vi "visualizer main.vi"(8 "error in (no error)":errorcluster, 11 "Item Ref in":T3 format="%.0x") -> (0 "error out":errorcluster, 3 "Item Ref out":T3 format="%.0x")   [LabVIEW 2016, in "FPGA RM System Definition API.lvlib"]
uses:
  FPGA RM System Definition API.lvlib
  <vilib>/NI Veristand/Custom Device API/Custom Device Item Ref.ctl
  API/Types/fpga resource.ctl
  API/Types/Channel Type.ctl
  type defs/viz_type.ctl
  type defs/viz_state.ctl
  visualizer globals.vi
  <vilib>/NI VeriStand/Custom Device Tools/Custom Device Utility Library/Custom Device Utility Library.lvlib
  Shared/FPGA RM Shared API.lvlib
  <vilib>/NI VeriStand/Custom Device API/Custom Device API.lvlib
panel:
  out "column width":i32[](array[numeric])
  in  "Options":enum32{"", "Sort", "Filter"}(tab)=enum."Filter"
  in  "Sort By...":T1 items=["RIO device", "resource", "input type", "datatype", "reserver"]
  in  "Datatype":string
  in  "Input Type":T2(ring)
  in  "Resource Name":string
  in  "RIO Device Name":string
  in  "Mappings":i32(listbox)
  in  "Columns":i32(listbox)
  out "mapped and unmapped":bool[](array[boolean])
  out "selected values":bool[](array[boolean])
  in  "table":i32(listbox)
  out "fpga resources":cluster{"fpga cd":T3, "resource":T4}[](array[cluster]) {"fpga cd" format="%.0x"}
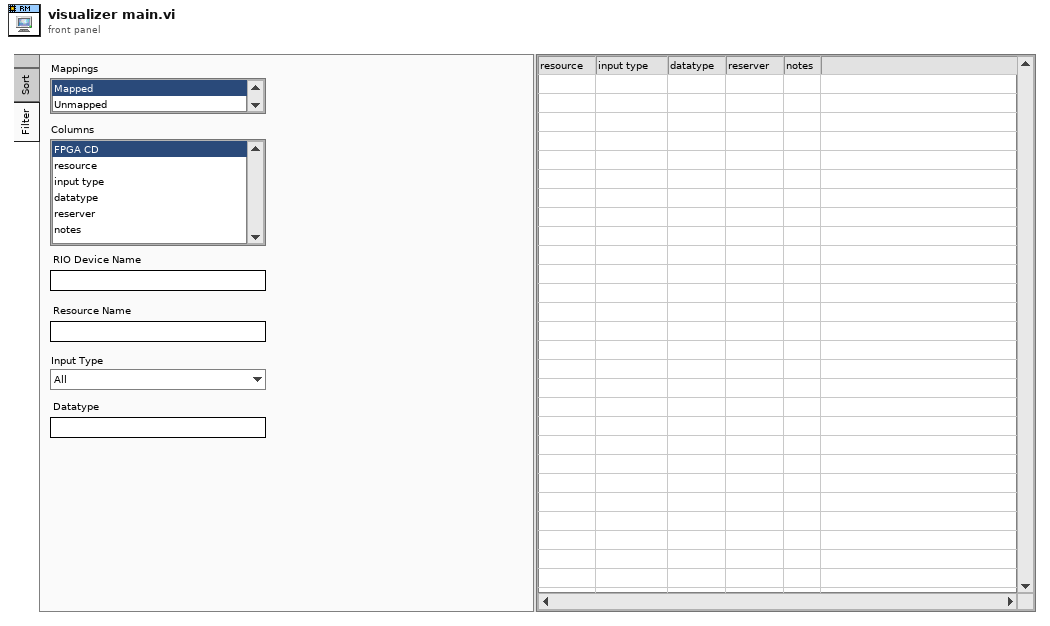
[diagram p1: front panel]
types:
  T1 = typedef "FPGA RM System Definition API.lvlib/viz_type.ctl" = u16
  T2 = enum16{"All", "Write Channel", "Read Channel", "Write Waveform", "Read Waveform"}
  T3 = typedef "Custom Device API.lvlib/Custom Device Item Ref.ctl" = u64
  T4 = typedef "FPGA RM System Definition API.lvlib/fpga resource.ctl" = cluster{"name":string, "datatype":string, "channel type":T5, "value":variant, "notes":string}
  T5 = typedef "FPGA RM System Definition API.lvlib/Channel Type.ctl" = enum16{"Write Channel", "Read Channel", "Write Waveform", "Read Waveform"}
  T6 = typedef "RM.Server.lvlib/viz_command.ctl" = cluster{"state":T7, "data":variant}
  T7 = typedef "RM.Server.lvlib/viz_state.ctl" = enum16{"shutdown"}
  T8 = typedef "FPGA RM System Definition API.lvlib/viz_state.ctl" = enum16{"shutdown"}
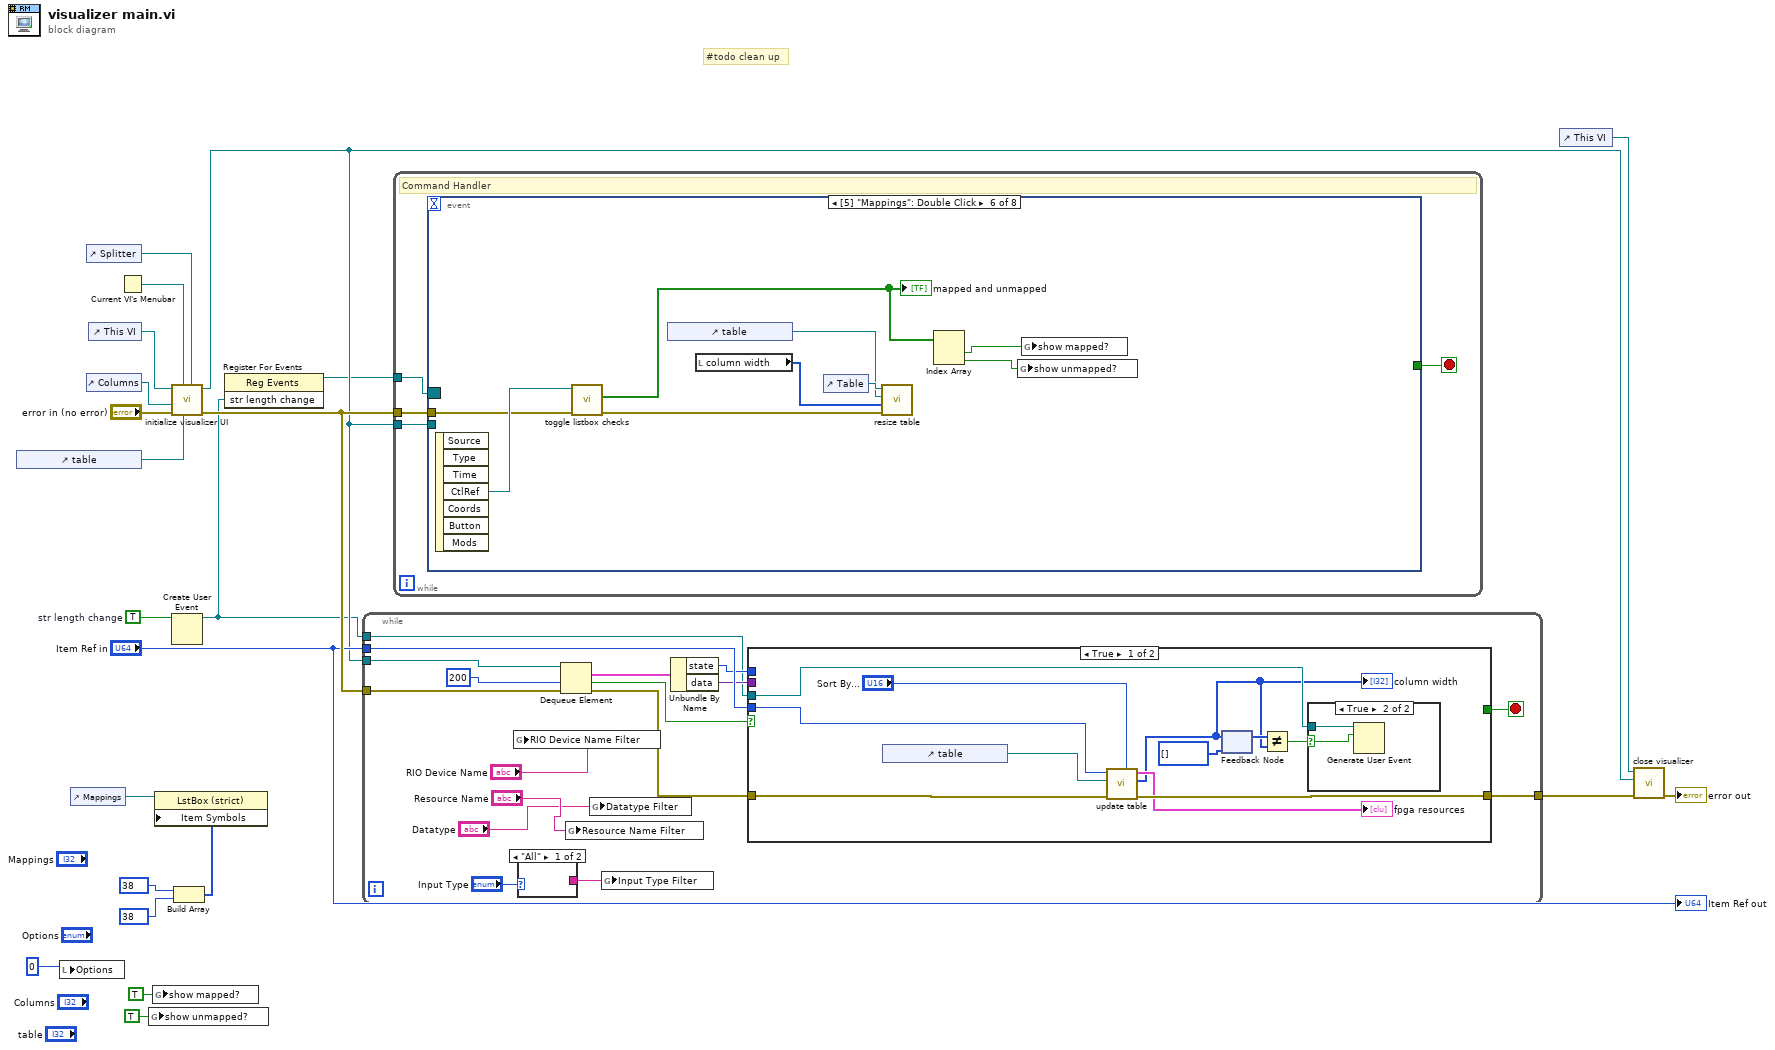
[diagram p0: block diagram]
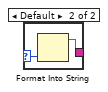
[diagram p2: hidden frame]
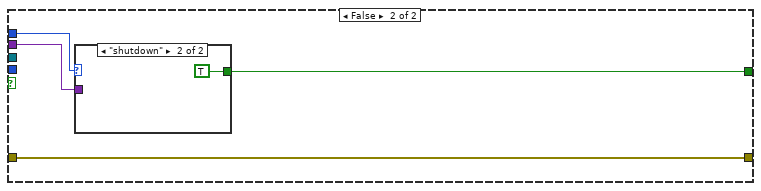
[diagram p4: hidden frame]
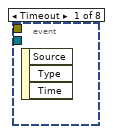
[diagram p6: hidden frame]
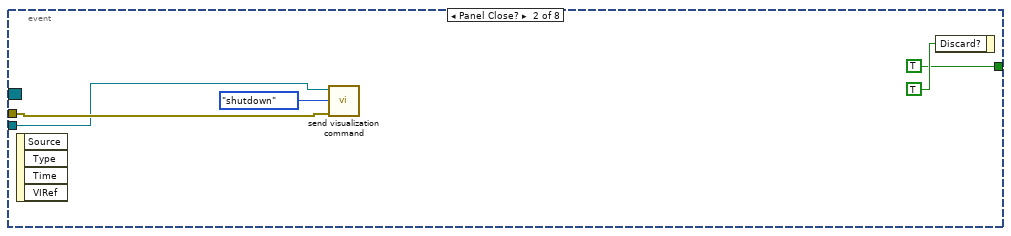
[diagram p7: hidden frame]
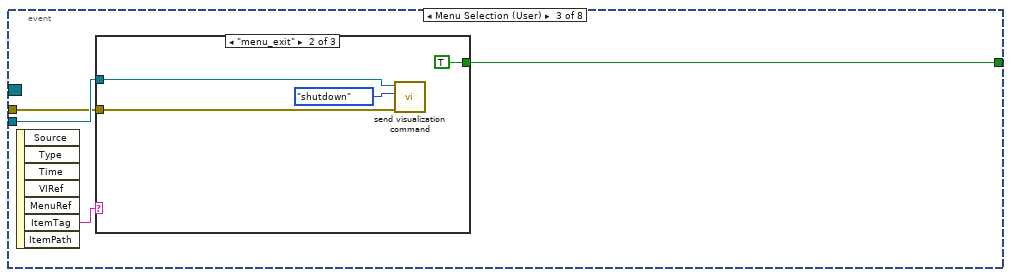
[diagram p8: hidden frame]
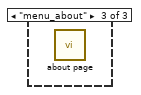
[diagram p10: hidden frame]
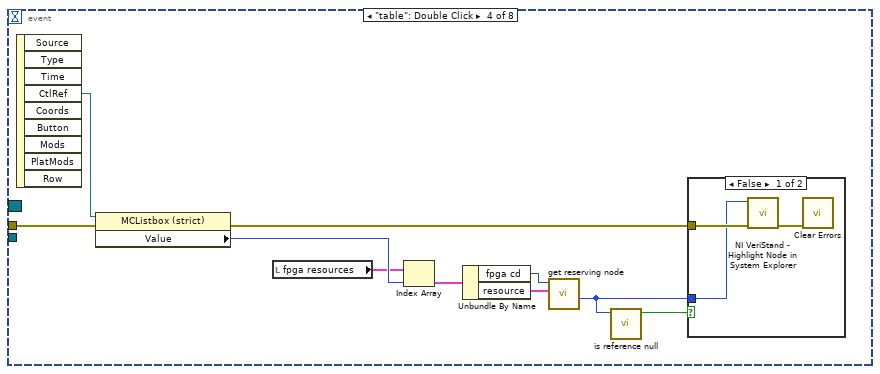
[diagram p11: hidden frame]
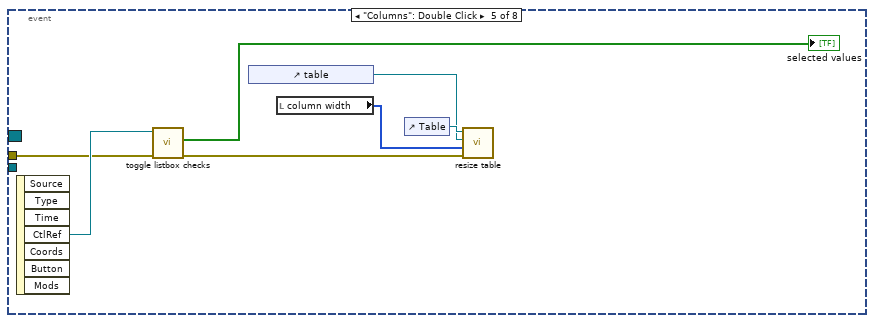
[diagram p13: hidden frame]
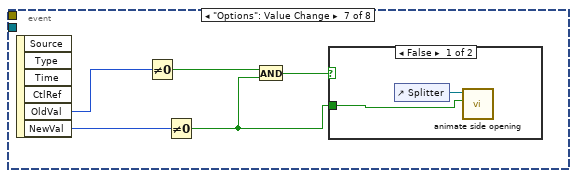
[diagram p14: hidden frame]
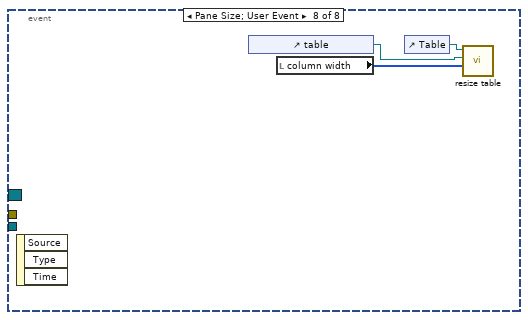
[diagram p16: hidden frame]
diagram:
  w10 = TRUE  # str length change
  # "#todo clean up"
  n1 = control-ref of="table"() -> (w12:refnum<vi>)
  n2 = local write "Options"(0) -> ()
  n3 = control-ref of="Mappings"() -> (w6:refnum<vi>)
  n4 = control-ref of="Splitter"() -> (w13:refnum<vi>)
  n5 = control-ref of="Columns"() -> (w11:refnum<vi>)
  n6 = control-ref of="This VI"() -> (w19:refnum<vi>)
  n7 = Current VI's Menubar() -> (w14:refnum<k9>)
  n8 = global write "visualizer globals.vi" "show unmapped?"(TRUE ("show unmapped?")) -> ()
  n9 = global write "visualizer globals.vi" "show mapped?"(TRUE ("show mapped?")) -> ()
  n10 = call "initialize visualizer UI.vi"("Splitter"=w13, "MCLB Reference"=w12, "menu reference in"=w14, "error in (no error)"="error in (no error)", "display"=w11, "VI in"=w19) -> ("error out"=w21:errorcluster, "Queue out"=w15:refnum<queue>)  [unwired: 4 in]
  n11 = Create User Event(user event datatype=w10) -> (user event=w8:refnum<user-event>)  [unwired: 1 in, 1 out]
  n12 = Build Array(38, 38) -> (w3:i32[])
  n13 = property class="LstBox (strict)"(reference=w6, "Item Symbols"=w3) -> ()  [unwired: 1 in, 2 out]
  n14 = register-events(w8) -> (reference out=w9:refnum<event-registration>)  [unwired: 2 in, 1 out]
  n15 = while {
    tunnel: w15 -> [w39]
    tunnel: w21 -> [w36]
    tunnel: "Item Ref in" -> [w34]
    tunnel: [w33] -> w18
    tunnel: w8 -> [w28]
    stop <- w37 stop-if-true
    n16 = global write "visualizer globals.vi" "RIO Device Name Filter"("RIO Device Name") -> ()
    n17 = case shown="\"All\"" "Input Type" {
      selector: "Input Type" -> [_ w41]
      tunnel: [_ w40] -> w24
      frame "All" {
      }
      frame Default {
        n18 = Format Into String(w41) -> (resulting string=w40:string)  [unwired: 3 in, 1 out]
      }
    }
    n19 = Dequeue Element(queue=w39, timeout in ms (-1)=200, error in (no error)=w36) -> (element=w38:T6, timed out?=w31:bool, error out=w35:errorcluster)  [unwired: 1 out]
    n20 = global write "visualizer globals.vi" "Resource Name Filter"("Resource Name") -> ()
    n21 = global write "visualizer globals.vi" "Datatype Filter"("Datatype") -> ()
    n22 = global write "visualizer globals.vi" "Input Type Filter"(w24) -> ()
    n23 = Unbundle By Name(w38) -> ("state"=w30:T7, "data"=w29:variant)
    n24 = case shown="True" w31 {
      tunnel: [_ w58] -> w37
      tunnel: w35 -> [w52 w57]
      tunnel: w34 -> [w49 _]
      tunnel: [w51 w57] -> w33
      tunnel: w30 -> [_ w56]
      tunnel: w29 -> [_ w55]
      tunnel: w28 -> [w45 _]
      frame True {
        n25 = control-ref of="table"() -> (w50:refnum<vi>)
        n26 = call "update table.vi"("Sort By..."="Sort By...", "error in (no error)"=w52, "MulticolumnListbox in"=w50, "Item Ref in"=w49) -> ("error out"=w51:errorcluster, "max string length in columns"=w43:i32[], "fpga resources out"=→"fpga resources":cluster{"fpga cd":T3, "resource":T4}[])  [unwired: 5 in]
        "column width" <- w43
        n27 = feedback-in #1(w43) -> ()
        n28 = feedback #1(i32[] [] ("max string length in columns")) -> (w46:i32[])
        n29 = Not Equal?(x=w46, y=w43) -> (x != y?=w44:bool)
        n30 = case shown="True" w44 {
          selector: w44 -> [_ w53]
          tunnel: w45 -> [_ w54]
          frame False {
          }
          frame True {
            n31 = Generate User Event(user event=w54, event data cluster=w53) -> ()  [unwired: 2 in, 2 out]
          }
        }
      }
      frame False {
        n32 = case shown="\"shutdown\"" w56 {
          tunnel: [_ TRUE] -> w58
          tunnel: w55 -> [_ _]
          frame Default {
          }
          frame "shutdown" {
          }
        }
      }
    }
  }
  n33 = while {
    tunnel: w15 -> [w62]
    tunnel: w21 -> [w61]
    tunnel: w9 -> [w60]
    stop <- w63 stop-if-true
    # "Command Handler"
    n34 = event shown="[5] \"Mappings\": Double Click" {
      selector: w60 -> [_ _ _ _ _ _ _ _]
      dyn-events: _ -> [_ _ _ _ _ _ _ _]
      timeout: _ -> [_ _ _ _ _ _ _ _]
      tunnel: [_ TRUE w71 _ _ _ _ _] -> w63
      tunnel: w62 -> [_ w64 w70 _ _ _ _ _]
      tunnel: w61 -> [_ w65 w69 w85 w95 w104 _ _]
      event Timeout {
        n35 = event-data() -> ()  [unwired: 1 in, 3 out]
      }
      event Panel Close? {
        n36 = event-data() -> ()  [unwired: 1 in, 4 out]
        n37 = call "send visualization command.vi"("error in (no error)"=w65, "state"=viz_state."shutdown" ("viz_state"), "Queue in"=w64) -> ()  [unwired: 8 in, 1 out]
        n38 = event-data("Discard?"=TRUE ("SilentShutdown")) -> ()  [unwired: 1 in, 1 out]
      }
      event Menu Selection (User) {
        n39 = event-data() -> ("ItemTag"=w72:string)  [unwired: 1 in, 6 out]
        n40 = case shown="\"menu_exit\"" w72 {
          tunnel: [_ TRUE _] -> w71
          tunnel: w70 -> [_ w75 _]
          tunnel: w69 -> [_ w73 _]
          frame Default {
          }
          frame "menu_exit" {
            n41 = call "send visualization command.vi"("error in (no error)"=w73, "state"=viz_state."shutdown" ("viz_state"), "Queue in"=w75) -> ()  [unwired: 8 in, 1 out]
          }
          frame "menu_about" {
            n42 = call "about page.vi"() -> ()  [unwired: 12 in]
          }
        }
      }
      event "table": Double Click {
        n43 = event-data() -> ("CtlRef"=w86:refnum<vi>)  [unwired: 1 in, 8 out]
        n44 = property class="MCListbox (strict)"(reference=w86, error in=w85) -> (error out=w83:errorcluster, "Value"=w84:i32)  [unwired: 1 out]
        n45 = local read "fpga resources"() -> (w82:cluster{"fpga cd":T3, "resource":T4}[])
        n46 = Index Array(array=w82, index=w84) -> (element=w79:cluster{"fpga cd":T3, "resource":T4})
        n47 = Unbundle By Name(w79) -> ("fpga cd"=w80:T3, "resource"=w78:T4)
        n48 = call "get reserving node.vi"("FPGA Resource"=w78, "Item Ref in"=w80) -> ("Dependent Node Ref"=w77:T3)  [unwired: 6 in, 3 out]
        n49 = call "is reference null.vi"("reserver"=w77) -> ("Boolean"=w81:bool)  [unwired: 10 in]
        n50 = case shown="False" w81 {
          tunnel: w83 -> [w89 _]
          tunnel: w77 -> [w88 _]
          frame False {
            n51 = call <vilib>:"NI VeriStand - Highlight Node in System Explorer.vi"("error in (no error)"=w89, "Item Ref in"=w88) -> ("error out"=w87:errorcluster)  [unwired: 8 in, 1 out]
            n52 = call <vilib>:"Clear Errors.vi"("error in (no error)"=w87) -> ()  [unwired: 5 in, 2 out]
          }
          frame True {
          }
        }
      }
      event "Columns": Double Click {
        n53 = event-data() -> ("CtlRef"=w96:refnum<vi>)  [unwired: 1 in, 6 out]
        n54 = call "toggle listbox checks.vi"("error in (no error)"=w95, "ListBox in"=w96) -> ("error out"=w91:errorcluster, "selected values"=→"selected values":bool[])  [unwired: 8 in]
        n55 = control-ref of="table"() -> (w93:refnum<vi>)
        n56 = local read "column width"() -> (w92:i32[])
        n57 = control-ref of="Table"() -> (w94:refnum<vi>)
        n58 = call "resize table.vi"("error in (no error)"=w91, "Column Weights"=w92, "table"=w93, "Pane in"=w94) -> ()  [unwired: 7 in, 1 out]
      }
      event "Mappings": Double Click {
        n59 = event-data() -> ("CtlRef"=w105:refnum<vi>)  [unwired: 1 in, 6 out]
        n60 = call "toggle listbox checks.vi"("error in (no error)"=w104, "ListBox in"=w105) -> ("error out"=w100:errorcluster, "selected values"=w99:bool[])  [unwired: 8 in]
        "mapped and unmapped" <- w99
        n61 = control-ref of="table"() -> (w102:refnum<vi>)
        n62 = local read "column width"() -> (w101:i32[])
        n63 = control-ref of="Table"() -> (w103:refnum<vi>)
        n64 = call "resize table.vi"("error in (no error)"=w100, "Column Weights"=w101, "table"=w102, "Pane in"=w103) -> ()  [unwired: 7 in, 1 out]
        n65 = Index Array(array=w99) -> (element #1=w98:bool, element #2=w97:bool)  [unwired: 2 in]
        n66 = global write "visualizer globals.vi" "show unmapped?"(w97) -> ()
        n67 = global write "visualizer globals.vi" "show mapped?"(w98) -> ()
      }
      event "Options": Value Change {
        n68 = event-data() -> ("OldVal"=w109:enum32{"", "Sort", "Filter"}, "NewVal"=w110:enum32{"", "Sort", "Filter"})  [unwired: 1 in, 4 out]
        n69 = Not Equal To 0?(x=w109) -> (x != 0?=w108:bool)
        n70 = Not Equal To 0?(x=w110) -> (x != 0?=w107:bool)
        n71 = And(x=w108, y=w107) -> (x .and. y?=w106:bool)
        n72 = case shown="False" w106 {
          tunnel: w107 -> [w111 _]
          frame False {
            n73 = control-ref of="Splitter"() -> (w112:refnum<vi>)
            n74 = call "animate side opening.vi"("expand/collapse"=w111, "Splitter in"=w112) -> ()  [unwired: 10 in]
          }
          frame True {
          }
        }
      }
      event Pane Size; User Event {
        n75 = event-data() -> ()  [unwired: 1 in, 3 out]
        n76 = control-ref of="table"() -> (w114:refnum<vi>)
        n77 = local read "column width"() -> (w113:i32[])
        n78 = control-ref of="Table"() -> (w115:refnum<vi>)
        n79 = call "resize table.vi"("Column Weights"=w113, "table"=w114, "Pane in"=w115) -> ()  [unwired: 8 in, 1 out]
      }
    }
  }
  n80 = control-ref of="This VI"() -> (w16:refnum<vi>)
  n81 = call "close visualizer.vi"("error in (no error)"=w18, "Queue in"=w15, "reference"=w16) -> ("error out"=→"error out":errorcluster)  [unwired: 8 in]
  "Item Ref out" <- "Item Ref in"
